vi "Test MQTT-3.1.2-11.vi"(8 "error in (no error)":errorcluster) -> (0 "error out":errorcluster)   [LabVIEW 2013]
uses:
  source/Control Packets/CONNECT/ConnectFlags -- cluster.ctl
  source/Control Packets/CONNECT/CONNECT.lvclass
  <vilib>/addons/_JKI Toolkits/Caraya/classes/Test/Test.lvclass
  <vilib>/addons/_JKI Toolkits/Caraya/classes/Assert/Assert.lvclass
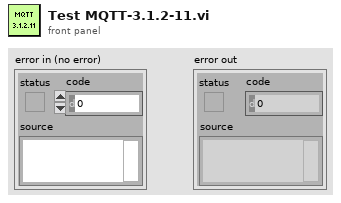
[diagram p1: front panel]
types:
  T1 = cluster{"Will Topic":string, "Will Message":string, "Username":string, "Password":string}
  T2 = typedef "CONNECT.lvclass/ConnectFlags -- cluster.ctl" = cluster{"Reserved":bool, "Clean Session":bool, "Will Flag":bool, "Will QoS 1":bool, "Will QoS 2":bool, "Will Retain":bool, "Password Flag":bool, "User Name Flag":bool}
  T3 = typedef "CONNECT.lvclass/ConnectPayload -- cluster.ctl" = cluster{"Will Topic":string, "Will Message":string, "Username":string, "Password":string}
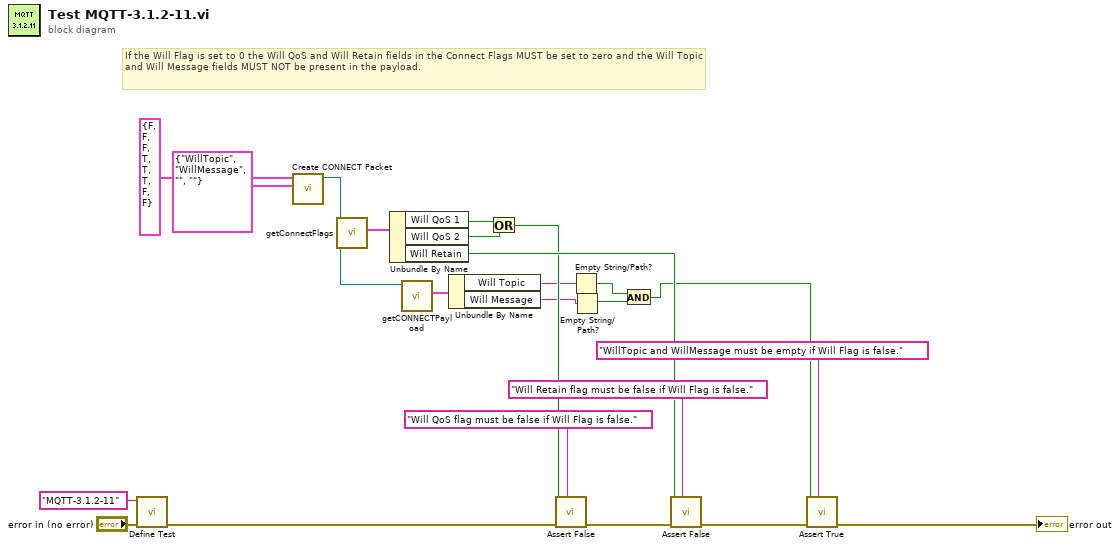
[diagram p0: block diagram]
diagram:
  # "If the Will Flag is set to 0 the Will QoS and Will Retain fields in the Connect Flags MUST be set to zero and the Will Topic and Will Message fields MUST NOT be present in the payload."
  n1 = call <vilib>:"Define Test.vi"("error in (no error)"="error in (no error)", "Label (VI Title)"="MQTT-3.1.2-11") -> ("error out"=w20:errorcluster)  [unwired: 9 in]
  n2 = call "Create CONNECT Packet.vi"("Payload"=T1 {"Will Topic"="WillTopic", "Will Message"="WillMessage", "Username"="", "Password"=""}, "Connect Flags"=T2 {"Reserved"=FALSE, "Clean Session"=FALSE, "Will Flag"=FALSE, "Will QoS 1"=TRUE, "Will QoS 2"=TRUE, "Will Retain"=TRUE, "Password Flag"=FALSE, "User Name Flag"=FALSE}) -> ("CONNECT"=w7:refnum<class "CONNECT.lvclass">)  [unwired: 8 in, 1 out]
  n3 = call "getConnectFlags.vi"("CONNECT in"=w7) -> ("Connect Flags"=w17:T2)  [unwired: 9 in, 1 out]
  n4 = Unbundle By Name(w17) -> ("Will QoS 1"=w16:bool, "Will QoS 2"=w8:bool, "Will Retain"=w13:bool)
  n5 = call "getCONNECTPayload.vi"("CONNECT in"=w7) -> ("Payload"=w6:T3)  [unwired: 9 in, 1 out]
  n6 = Unbundle By Name(w6) -> ("Will Topic"=w5:string, "Will Message"=w4:string)
  n7 = Or(x=w16, y=w8) -> (x .or. y?=w12:bool)
  n8 = call <vilib>:"Assert False.vi"("Label"="Will QoS flag must be false if Will Flag is false.", "error in (no error)"=w20, "False?"=w12) -> ("error out"=w15:errorcluster)  [unwired: 8 in]
  n9 = Empty String/Path?(string/path=w5) -> (empty?=w2:bool)
  n10 = Empty String/Path?(string/path=w4) -> (empty?=w3:bool)
  n11 = And(x=w2, y=w3) -> (x .and. y?=w1:bool)
  n12 = call <vilib>:"Assert False.vi"("Label"="Will Retain flag must be false if Will Flag is false.", "error in (no error)"=w15, "False?"=w13) -> ("error out"=w11:errorcluster)  [unwired: 8 in]
  n13 = call <vilib>:"Assert True.vi"("Label"="WillTopic and WillMessage must be empty if Will Flag is false.", "error in (no error)"=w11, "True?"=w1) -> ("error out"=→"error out":errorcluster)  [unwired: 8 in]
